vi "integrate.vi"(5 "waiting iterations per pixel":u32, 7 "integration iterations per pixel":u32, 9 "iteration counter in":u32, 10 "sampling values in":T1, 11 "previous pixel values in":T1) -> (1 "finished?":bool, 2 "iteration counter out":u32, 3 "new pixel values out":T1)   [LabVIEW 2010]
uses:
  common_typedefs/channels_cluster.ctl
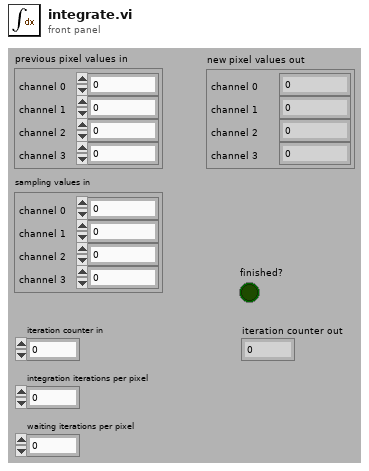
[diagram p1: front panel]
types:
  T1 = typedef "channels_cluster.ctl" = cluster{"channel 0":u32, "channel 1":u32, "channel 2":u32, "channel 3":u32}
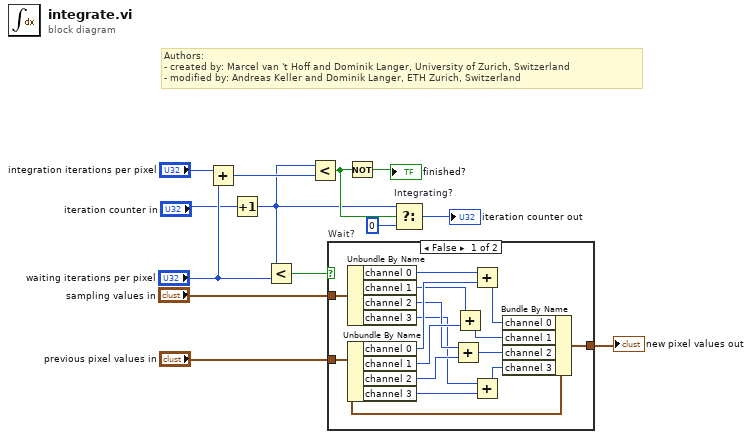
[diagram p0: block diagram]
diagram:
  # "Authors: \n- created by: Marcel van 't Hoff and Dominik Langer, University of Zurich, Switzerland\n- modified by: Andreas Keller and Dominik Langer, ETH Zurich, Switzerland"
  n1 = Add(x="integration iterations per pixel", y="waiting iterations per pixel") -> (x+y=w6:u32)
  n2 = Increment(x="iteration counter in") -> (x+1=w3:u32)
  n3 = Less?(x=w3, y="waiting iterations per pixel") -> (x < y?=w7:bool)
  n4 = Less?(x=w3, y=w6) -> (x < y?=w4:bool)
  n5 = case "Wait?" shown="False" w7 {
    tunnel: "sampling values in" -> [w20 _]
    tunnel: "previous pixel values in" -> [w19 w29]
    tunnel: [w14 w29] -> w11
    frame False {
      n6 = Unbundle By Name(w20) -> ("channel 0"=w28:u32, "channel 1"=w26:u32, "channel 2"=w24:u32, "channel 3"=w22:u32)
      n7 = Unbundle By Name(w19) -> ("channel 0"=w27:u32, "channel 1"=w25:u32, "channel 2"=w23:u32, "channel 3"=w21:u32)
      n8 = Add(x=w24, y=w23) -> (x+y=w16:u32)
      n9 = Add(x=w26, y=w25) -> (x+y=w17:u32)
      n10 = Add(x=w28, y=w27) -> (x+y=w18:u32)
      n11 = Add(x=w22, y=w21) -> (x+y=w15:u32)
      n12 = Bundle By Name(cluster=w19, "channel 0"=w18, "channel 1"=w17, "channel 2"=w16, "channel 3"=w15) -> (w14:T1)
    }
    frame True {
    }
  }
  "new pixel values out" <- w11
  n13 = Not(x=w4) -> (.not. x?=→"finished?":bool)
  n14 = Select "Integrating?"(t=w3, s=w4, f=u32 0) -> (s? t:f=→"iteration counter out":u32)
